vi "DataToSaveV2.vi"(7 "Logging Type":enum16{"Disable Log", "TDMS", "CSV"}(ring), 8 "error in (no error)":errorcluster, 10 "Message Queues out":T2, 11 "GlobalData":T1) -> (0 "error out":errorcluster)   [LabVIEW 2024]
doc: "This VI Send data to Logging loop to save"
uses:
  Message Queue/All Message Queues.ctl
  Message Queue/Message Cluster.ctl
  controls/GlobalData.ctl
  Message Queue/Enqueue Message (Single).vi
  Message Queue/Message Queue.lvlib
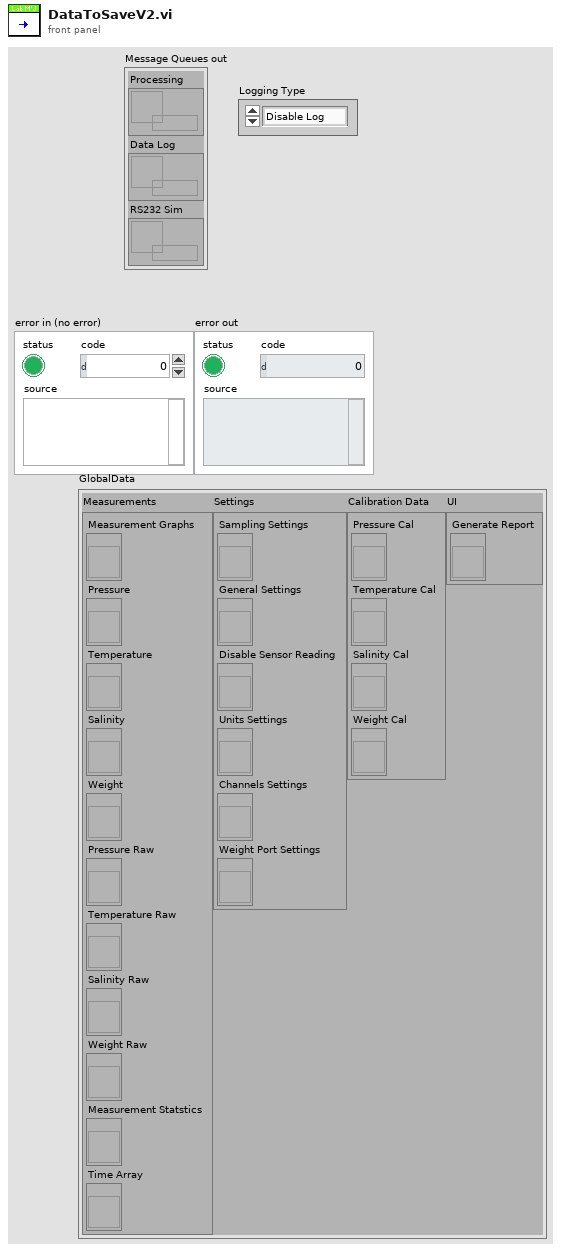
[diagram p1: front panel]
types:
  T1 = typedef "GlobalData.ctl" = cluster{"Measurements":cluster{"Measurement Graphs":refnum<vi>, "Pressure":refnum<vi>, "Temperature":refnum<vi>, "Salinity":refnum<vi>, "Weight":refnum<vi>, "Pressure Raw":refnum<vi>, "Temperature Raw":refnum<vi>, "Salinity Raw":refnum<vi>, "Weight Raw":refnum<vi>, "Measurement Statstics":refnum<vi>, "Time Array":refnum<vi>}, "Settings":cluster{"Sampling Settings":refnum<vi>, "General Settings":refnum<vi>, "Disable Sensor Reading":refnum<vi>, "Units Settings":refnum<vi>, "Channels Settings":refnum<vi>, "Weight Port Settings":refnum<vi>}, "Calibration Data":cluster{"Pressure Cal":refnum<vi>, "Temperature Cal":refnum<vi>, "Salinity Cal":refnum<vi>, "Weight Cal":refnum<vi>}, "UI":cluster{"Generate Report":refnum<vi>}}
  T2 = typedef "Message Queue.lvlib/All Message Queues.ctl" = cluster{"Processing":refnum<queue>, "Data Log":refnum<queue>, "RS232 Sim":refnum<queue>}
  T3 = cluster{"Pressure":dbl[], "Temperature":dbl[], "Salinity":dbl[], "Weight":dbl[]}
  T4 = cluster{"Reading Time (ms)":u64, "Graph Time ":u16}
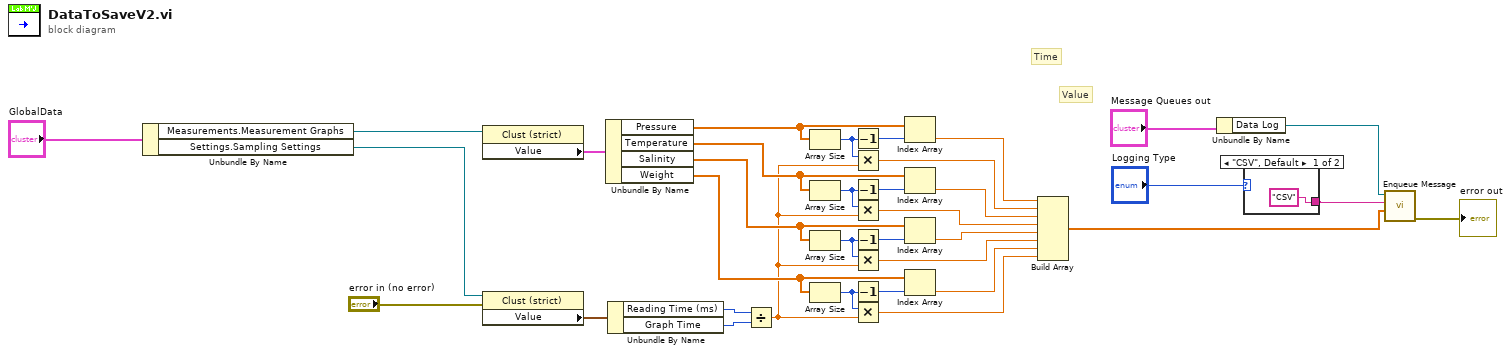
[diagram p0: block diagram]
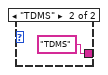
[diagram p2: hidden frame]
diagram:
  # "Time"
  # "Value"
  n1 = Unbundle By Name("GlobalData") -> ("Measurements.Measurement Graphs"=w34:refnum<vi>, "Settings.Sampling Settings"=w21:refnum<vi>)
  n2 = property on="Property Node" class="Clust (strict)"(reference=w34) -> ("Value"=w33:T3)  [unwired: 1 in, 2 out]
  n3 = property on="Property Node" class="Clust (strict)"(reference=w21, error in="error in (no error)") -> ("Value"=w20:T4)  [unwired: 2 out]
  n4 = Unbundle By Name(w33) -> ("Pressure"=w32:dbl[], "Temperature"=w28:dbl[], "Salinity"=w27:dbl[], "Weight"=w26:dbl[])
  n5 = Unbundle By Name(w20) -> ("Reading Time (ms)"=w17:u64, "Graph Time"=w19:u16)
  n6 = Divide(x=w17, y=w19) -> (x/y=w11:dbl)
  n7 = Array Size(array=w32) -> (size(s)=w18:i32)
  n8 = Array Size(array=w28) -> (size(s)=w14:i32)
  n9 = Array Size(array=w27) -> (size(s)=w13:i32)
  n10 = Array Size(array=w26) -> (size(s)=w12:i32)
  n11 = Decrement(x=w18) -> (x-1=w31:i32)
  n12 = Multiply(x=w18, y=w11) -> (x*y=w15:dbl)
  n13 = Decrement(x=w14) -> (x-1=w16:i32)
  n14 = Multiply(x=w14, y=w11) -> (x*y=w10:dbl)
  n15 = Decrement(x=w13) -> (x-1=w30:i32)
  n16 = Multiply(x=w13, y=w11) -> (x*y=w9:dbl)
  n17 = Decrement(x=w12) -> (x-1=w29:i32)
  n18 = Multiply(x=w12, y=w11) -> (x*y=w8:dbl)
  n19 = Index Array(array=w32, index=w31) -> (element=w25:dbl)
  n20 = Index Array(array=w28, index=w16) -> (element=w24:dbl)
  n21 = Index Array(array=w27, index=w30) -> (element=w23:dbl)
  n22 = Index Array(array=w26, index=w29) -> (element=w22:dbl)
  n23 = Build Array(w25, w15, w24, w10, w23, w9, w22, w8) -> (w6:dbl[])
  n24 = Unbundle By Name("Message Queues out") -> ("Data Log"=w7:refnum<queue>)
  n25 = case shown="\"CSV\", Default" "Logging Type" {
    tunnel: ["CSV" ("Message") "TDMS" ("Message")] -> w3
    frame "CSV", Default {
    }
    frame "TDMS" {
    }
  }
  n26 = call-poly "Enqueue Message.vi"("Message Data"=w6, "Message"=w3, "Message Queue"=w7) -> ("error out"=→"error out":errorcluster)  [unwired: 7 in, 1 out]
